vi "Read Icon.vi"(8 "error in (no error)":errorcluster, 11 "TTLDevice in":refnum<class "TCPControlledDevice.lvclass">) -> (0 "error out":errorcluster, 2 "Icon":picture, 3 "TTLDevice out":refnum<class "TCPControlledDevice.lvclass">)   [LabVIEW 2020, in "TCPControlledDevice.lvclass"]
uses:
  TCPControlledDevice.lvclass
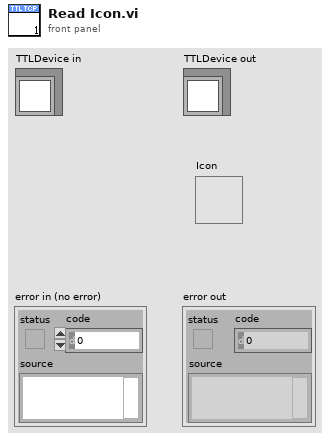
[diagram p1: front panel]
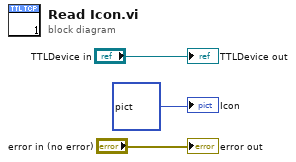
[diagram p0: block diagram]
diagram:
  "error out" <- "error in (no error)"
  "TTLDevice out" <- "TTLDevice in"
  "Icon" <- picture bytes[7230] ("new picture")
